vi "PH_SRDG645.get Output.vi"(0 "i ref in":refnum<vi>, 1 "Output BNC (T0)":T1 items=["T0", "AB", "CD", "EF", "GH"], 5 "error IO":errorcluster) -> (14 "i ref out":refnum<vi>, 19 "error out":errorcluster)   [LabVIEW 2014, in "PH_SRDG645.lvlib"]
doc: "This VI querries the outputl settings from the hardware."
uses:
  PH_SRDG645.lvlib
  PH_SRDG645.Output Settings.ctl
  instr.lib/SRDG645/Driver/Output BNC.ctl
  instr.lib/SRDG645/Driver/Polarity.ctl
  instr.lib/SRDG645/Stanford Research DG645 - Driver.lvlib
panel:
  in  "Output cluster":T2={"Level Offset [V]"=0.0, "Amplitue [V]"=1000.0, "Polarity"=0} {"Polarity" items=["negative", "positive"]}
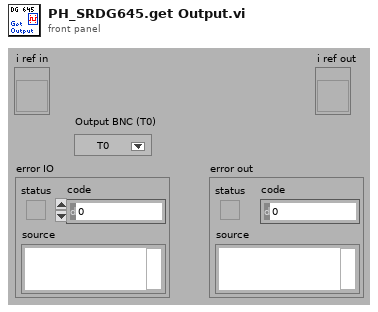
[diagram p1: front panel]
types:
  T1 = typedef "Stanford Research DG645 - Driver.lvlib/Output BNC.ctl" = i32
  T2 = typedef "PH_SRDG645.lvlib/PH_SRDG645.Output Settings.ctl" = cluster{"Level Offset [V]":dbl, "Amplitue [V]":dbl, "Polarity":i32}
  T3 = typedef "PH_SRDG645.lvlib/PH_SRDG645.i attribute.ctl" = cluster{"GUI Refs":cluster{"Delete":refnum<vi>, "Device Errors":refnum<vi>, "Trigger":refnum<vi>, "Default Name":refnum<vi>, "Firmware Revision":refnum<vi>, "Serial Number":refnum<vi>, "Model":refnum<vi>, "Visa resource name":refnum<vi>}, "Service ID Rate":i32, "Service IDs Channelinfo":i32[], "VISA resource name":refnum<visa-resource-name>, "Device Errors":cluster{"code":i32, "Text":string}[], "Trigger":T4, "Channels":cluster{"T1":T5, "A":T5, "B":T5, "C":T5, "D":T5, "E":T5, "F":T5, "G":T5, "H":T5}, "GUI Refs Channels":refnum<vi>[], "Outputs":cluster{"AB":cluster{"Level Offset [V]":dbl, "Amplitue [V]":dbl, "Polarity":i32}, "CD":cluster{"Level Offset [V]":dbl, "Amplitue [V]":dbl, "Polarity":i32}, "EF":cluster{"Level Offset [V]":dbl, "Amplitue [V]":dbl, "Polarity":i32}, "GH":cluster{"Level Offset [V]":dbl, "Amplitue [V]":dbl, "Polarity":i32}, "T0":cluster{"Level Offset [V]":dbl, "Amplitue [V]":dbl, "Polarity":i32}}, "GUI Refs Outputs":refnum<vi>[], "Serial Number":string, "Firmweare Revision":string, "Model":string}
  T4 = typedef "PH_SRDG645.lvlib/PH_SRDG645.Trigger.ctl" = cluster{"Source":i32, "Rate [Hz]":dbl, "Level [V]":dbl}
  T5 = typedef "PH_SRDG645.lvlib/PH_SRDG645.Channel Settings.ctl" = cluster{"Delay [s]":dbl, "relative to":i32}
  T6 = typedef "Stanford Research DG645 - Driver.lvlib/Polarity.ctl" = i32
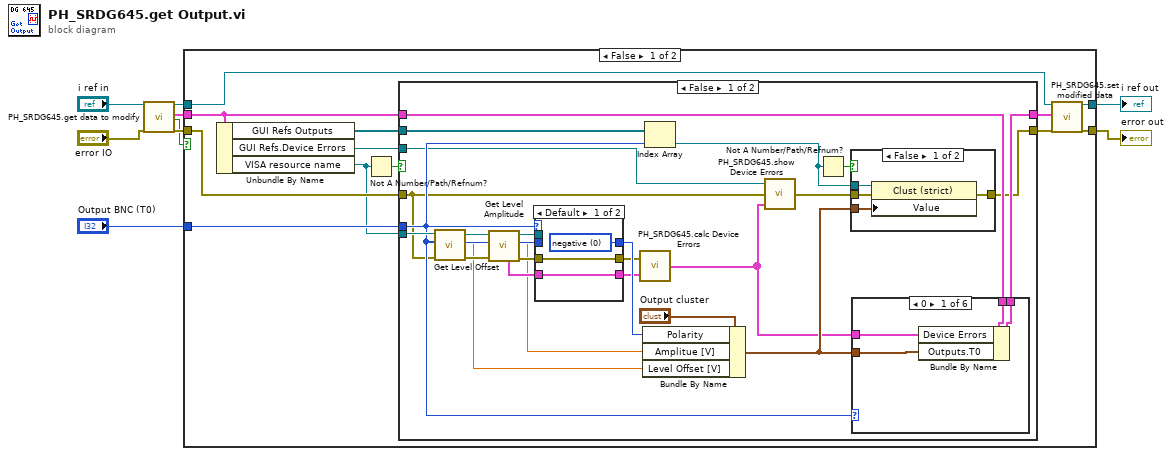
[diagram p0: block diagram]
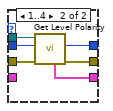
[diagram p2: hidden frame]
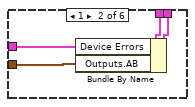
[diagram p3: hidden frame]
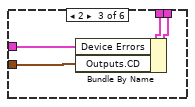
[diagram p4: hidden frame]
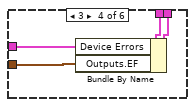
[diagram p5: hidden frame]
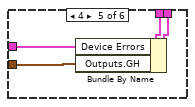
[diagram p6: hidden frame]
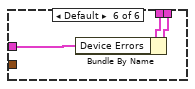
[diagram p7: hidden frame]
diagram:
  n1 = call "PH_SRDG645.get data to modify.vi"("i ref in"="i ref in", "error in (no error)"="error IO") -> ("i ref out"=w7:refnum<vi>, "i attribute"=w4:T3, "timed out"=w2:bool, "error out"=w5:errorcluster)  [unwired: 14 in]
  n2 = case shown="False" w2 {
    tunnel: w7 -> [w12 w86]
    tunnel: [w21 w86] -> w6
    tunnel: w5 -> [w14 w85]
    tunnel: w4 -> [w20 _]
    tunnel: [w18 w85] -> w3
    tunnel: "Output BNC (T0)" -> [w13 _]
    frame False {
      n3 = Unbundle By Name(w20) -> ("GUI Refs Outputs"=w16:refnum<vi>[], "GUI Refs.Device Errors"=w15:refnum<vi>, "VISA resource name"=w10:refnum<visa-resource-name>)
      n4 = Not A Number/Path/Refnum?(number/path/refnum=w10) -> (NaN/Path/Refnum?=w11:bool)
      n5 = case shown="False" w11 {
        tunnel: w20 -> [w44 w84]
        tunnel: [w43 w84] -> w19
        tunnel: [w42 w83] -> w17
        tunnel: w16 -> [w40 _]
        tunnel: w15 -> [w30 _]
        tunnel: w14 -> [w22 w83]
        tunnel: w10 -> [w35 _]
        tunnel: w13 -> [w32 _]
        frame False {
          n6 = call "Get Level Offset.vi"("error in (no error)"=w22, "Output BNC (T0)"=w32, "VISA resource name"=w35) -> ("error out"=w36:errorcluster, "Level Offset [V]"=w27:dbl, "VISA resource name out"=w34:refnum<visa-resource-name>)  [unwired: 5 in, 1 out]
          n7 = call "Get Level Amplitude.vi"("error in (no error)"=w36, "Output BNC (T0)"=w32, "VISA resource name"=w34) -> ("error out"=w37:errorcluster, "Level Amplitue [V]"=w28:dbl, "VISA resource name out"=w33:refnum<visa-resource-name>, "Device Errors"=w31:cluster{"code":i32, "Text":string}[])  [unwired: 5 in]
          n8 = case shown="Default" w32 {
            tunnel: w37 -> [w48 w54]
            tunnel: [w46 w53] -> w23
            tunnel: [w48 w52] -> w25
            tunnel: w33 -> [_ w51]
            tunnel: w32 -> [_ w50]
            tunnel: [w47 w49] -> w26
            tunnel: w31 -> [w46 _]
            frame Default {
              w47 = T6 0 items=["negative", "positive"] ("Polarity")
            }
            frame 1..4 {
              n9 = call "Get Level Polarity.vi"("error in (no error)"=w54, "Output BNC (AB)"=w50, "VISA resource name"=w51) -> ("error out"=w52:errorcluster, "Polarity"=w49:T6, "Device Errors"=w53:cluster{"code":i32, "Text":string}[])  [unwired: 5 in, 1 out]
            }
          }
          n10 = call "PH_SRDG645.calc Device Errors.vi"("Device Errors out"=w23, "SRDG 645 error out"=w25) -> ("calculate Device Errors"=w24:cluster{"code":i32, "Text":string}[])
          n11 = Bundle By Name(cluster="Output cluster", "Polarity"=w26, "Amplitue [V]"=w28, "Level Offset [V]"=w27) -> (w38:T2)
          n12 = Index Array(array=w40, index=w32) -> (element=w39:refnum<vi>)
          n13 = call "PH_SRDG645.show Device Errors.vi"("Device Errors"=w24, "error in"=w22, "Ref Device Errors"=w30) -> ("error out"=w29:errorcluster)
          n14 = Not A Number/Path/Refnum?(number/path/refnum=w39) -> (NaN/Path/Refnum?=w41:bool)
          n15 = case shown="False" w41 {
            tunnel: w39 -> [w81 _]
            tunnel: w38 -> [w80 _]
            tunnel: w29 -> [w79 w82]
            tunnel: [w78 w82] -> w42
            frame False {
              n16 = property class="Clust (strict)"(reference=w81, error in=w79, "Value"=w80) -> (error out=w78:errorcluster)  [unwired: 1 out]
            }
            frame True {
            }
          }
          n17 = case shown="0" w32 {
            tunnel: w44 -> [w58 w62 w66 w70 w74 w77]
            tunnel: [w56 w61 w65 w69 w73 w76] -> w43
            tunnel: w38 -> [w55 w59 w63 w67 w71 _]
            tunnel: w24 -> [w57 w60 w64 w68 w72 w75]
            frame 0 {
              n18 = Bundle By Name(cluster=w58, "Device Errors"=w57, "Outputs.T0"=w55) -> (w56:T3)
            }
            frame 1 {
              n19 = Bundle By Name(cluster=w62, "Device Errors"=w60, "Outputs.AB"=w59) -> (w61:T3)
            }
            frame 2 {
              n20 = Bundle By Name(cluster=w66, "Device Errors"=w64, "Outputs.CD"=w63) -> (w65:T3)
            }
            frame 3 {
              n21 = Bundle By Name(cluster=w70, "Device Errors"=w68, "Outputs.EF"=w67) -> (w69:T3)
            }
            frame 4 {
              n22 = Bundle By Name(cluster=w74, "Device Errors"=w72, "Outputs.GH"=w71) -> (w73:T3)
            }
            frame Default {
              n23 = Bundle By Name(cluster=w77, "Device Errors"=w75) -> (w76:T3)
            }
          }
        }
        frame True {
        }
      }
      n24 = call "PH_SRDG645.set modified data.vi"("i ref in"=w12, "i attribute"=w19, "error in (no error)"=w17) -> ("i ref out"=w21:refnum<vi>, "error out"=w18:errorcluster)  [unwired: 15 in]
    }
    frame True {
    }
  }
  "error out" <- w3
  "i ref out" <- w6
